vi "Swap A and B.vi"() -> ()   [LabVIEW 2009]
panel:
  out "B":u32
  out "A":u32
  out "AXorB":bool[](array[boolean])
  out "B=(AXorB)XorB":bool[](array[boolean])
  out "A=((AXorB)XorB)Xor(AXorB)":bool[](array[boolean])
  out "Boolean array number B":bool[](array[boolean])
  out "Boolean array number A":bool[](array[boolean])
  in  "number B":u32
  in  "number A":u32
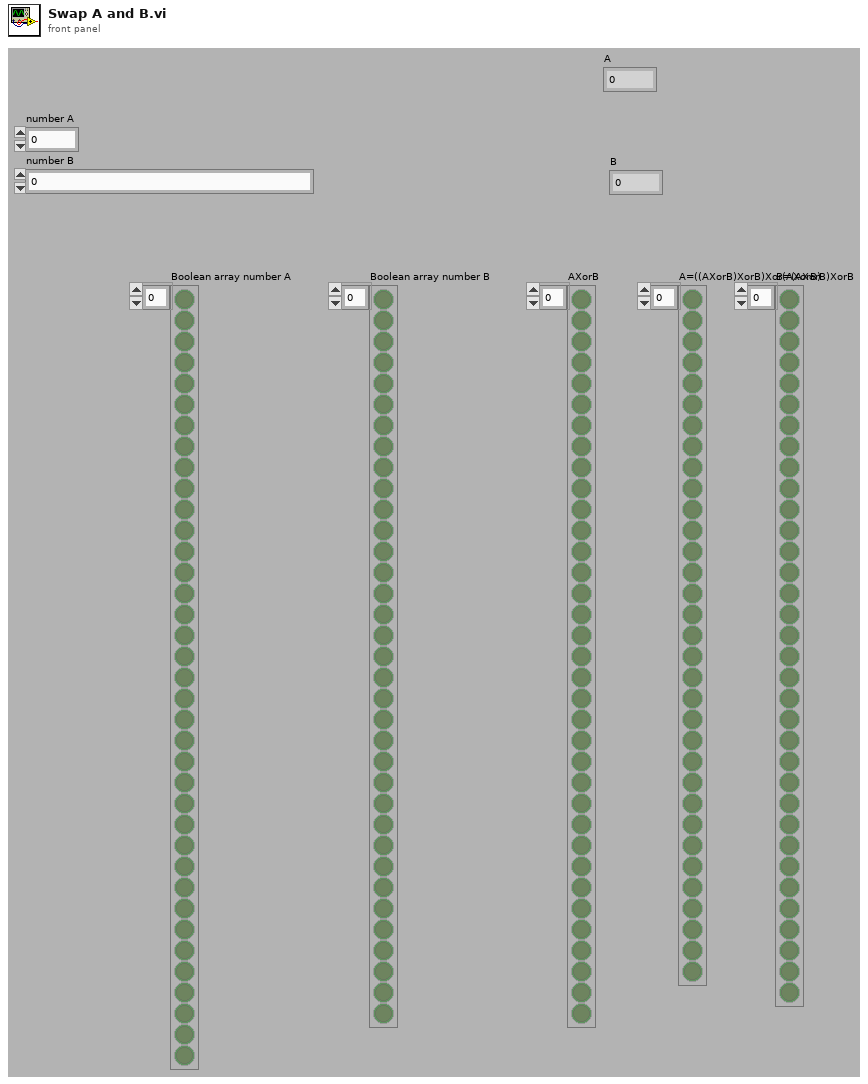
[diagram p1: front panel]
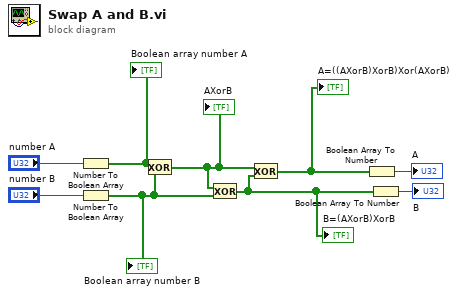
[diagram p0: block diagram]
diagram:
  n1 = Number To Boolean Array(number="number A") -> (Boolean array=w7:bool[])
  "Boolean array number A" <- w7
  n2 = Number To Boolean Array(number="number B") -> (Boolean array=w6:bool[])
  "Boolean array number B" <- w6
  n3 = Exclusive Or(1:w6, 2:w7) -> (0:w5:bool[])
  "AXorB" <- w5
  n4 = Exclusive Or(1:w6, 2:w5) -> (0:w1:bool[])
  "B=(AXorB)XorB" <- w1
  n5 = Exclusive Or(1:w1, 2:w5) -> (0:w4:bool[])
  "A=((AXorB)XorB)Xor(AXorB)" <- w4
  n6 = Boolean Array To Number(Boolean array=w4) -> (number=→"A":u32)
  n7 = Boolean Array To Number(Boolean array=w1) -> (number=→"B":u32)
